vi "List Contents of Azure Container.vi"() -> ()   [LabVIEW 2015]
doc: "Demonstrates how to display the contents of a container for the Azure Blob Service."
uses:
  Core/Azure Credentials.ctl
  Core/NI_Azure_Core.lvlib
  Core/Session/Session.lvclass
  Blob Storage/NI_Azure_Blob.lvlib
panel:
  in  "Access Key":string
  in  "Container Name":string
  in  "Storage Account Name":string
  out "Container Contents":i32(listbox)
  # "Overview: Demonstrates how to display the contents of a container for the Azure Blob Service.\nRequirements: NI Cloud Toolkit for Azure and a registered Microsoft Azure account\nInstructions:\n1. Specify the Storage Account Name and Access Key for your Azure account. You can create an account at http://azure.microsoft.com.\n2. Specify a Container Name for the container you want to inspect.\n3. Run the VI. All of the contents of the specified container will be displayed in the Container Contents indicator."
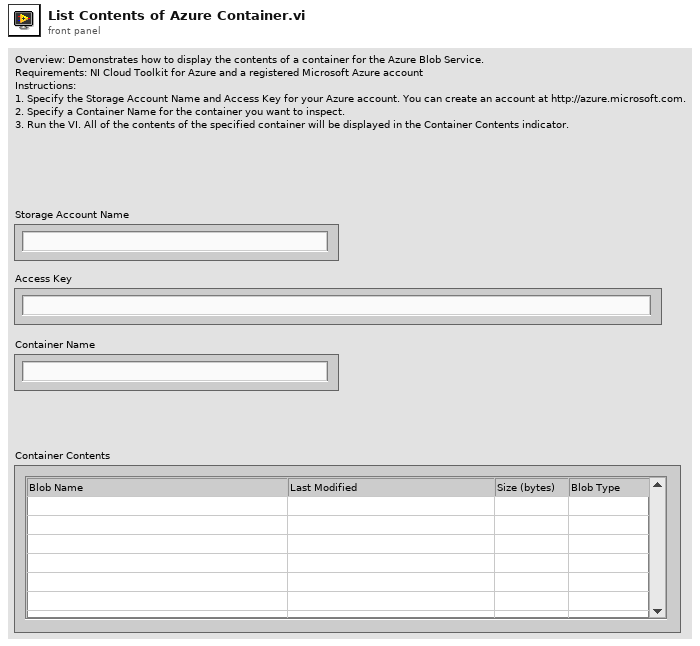
[diagram p1: front panel]
types:
  T1 = typedef "NI_Azure_Core.lvlib/Azure Credentials.ctl" = cluster{"Storage Account Name":string, "Access Key":string}
  T2 = typedef "NI_Azure_Core.lvlib/Name Value Pair.ctl" = cluster{"name":string, "value":string}
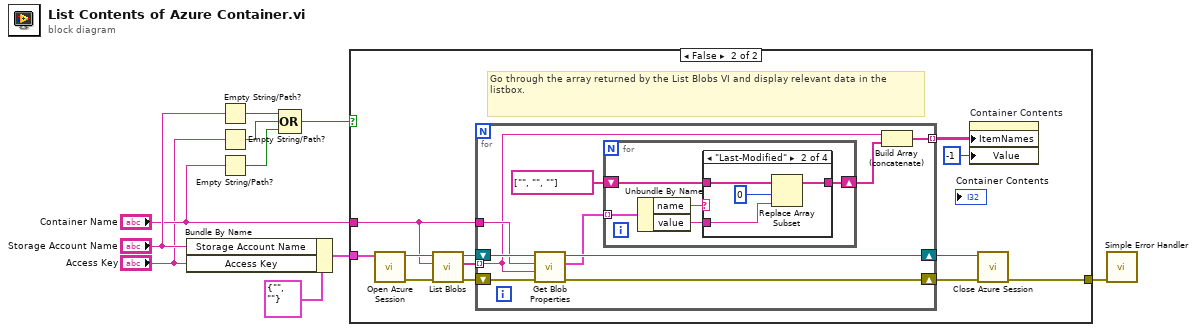
[diagram p0: block diagram]
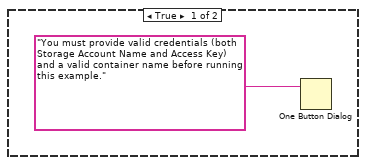
[diagram p2: hidden frame]
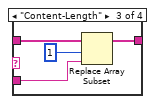
[diagram p4: hidden frame]
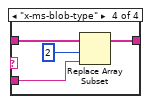
[diagram p5: hidden frame]
diagram:
  n1 = Bundle By Name(cluster=T1 {"Storage Account Name"="", "Access Key"=""} ("Credentials"), "Storage Account Name"="Storage Account Name", "Access Key"="Access Key") -> (w3:T1)
  n2 = Empty String/Path?(string/path="Storage Account Name") -> (empty?=w10:bool)
  n3 = Empty String/Path?(string/path="Access Key") -> (empty?=w9:bool)
  n4 = Empty String/Path?(string/path="Container Name") -> (empty?=w4:bool)
  n5 = Compound Arithmetic op=OR(w10, w9, w4) -> (w7:bool)
  n6 = case shown="False" w7 {
    tunnel: w3 -> [_ w23]
    tunnel: [_ w16] -> w6
    tunnel: "Container Name" -> [_ w14]
    frame True {
      n7 = One Button Dialog(message="You must provide valid credentials (both Storage Account Name and Access Key) and a valid container name before running this example.") -> ()  [unwired: 1 in, 1 out]
    }
    frame False {
      # "Go through the array returned by the List Blobs VI and display relevant data in the listbox."
      n8 = call "Open Azure Session.vi"("Credentials"=w23) -> ("error out"=w22:errorcluster, "Azure Session"=w21:refnum<class "Session.lvclass">)  [unwired: 9 in]
      n9 = call "List Blobs.vi"("error in (no error)"=w22, "Container"=w14, "Azure Session in"=w21) -> ("error out"=w20:errorcluster, "Blobs"=w15:string[], "Azure Session out"=w19:refnum<class "Session.lvclass">)  [unwired: 6 in]
      n10 = for {
        tunnel: w15 -> [w28] mode=indexing
        shift-right: [w29] -> w17
        shift-left: w20 -> [w33]
        shift-right: [w30] -> w18
        shift-left: w19 -> [w32]
        tunnel: w14 -> [w31]
        tunnel: [w27] -> w13 mode=indexing
        n11 = call "Get Blob Properties.vi"("error in (no error)"=w33, "Blob"=w28, "Container"=w31, "Azure Session in"=w32) -> ("error out"=w29:errorcluster, "Blob Properties"=w26:T2[], "Azure Session out"=w30:refnum<class "Session.lvclass">)  [unwired: 5 in]
        n12 = for {
          tunnel: w26 -> [w38] mode=indexing
          shift-right: [w34] -> w25
          shift-left: string[] ["", "", ""] -> [w35]
          n13 = Unbundle By Name(w38) -> ("name"=w37:string, "value"=w36:string)
          n14 = case shown="\"Last-Modified\"" w37 {
            tunnel: w36 -> [_ w41 w45 w49]
            tunnel: w35 -> [w39 w43 w47 w51]
            tunnel: [w39 w42 w46 w50] -> w34
            frame Default {
            }
            frame "Last-Modified" {
              n15 = Replace Array Subset(array=w43, new element=w41, index=0) -> (w42:string[])
            }
            frame "Content-Length" {
              n16 = Replace Array Subset(array=w47, new element=w45, index=1) -> (w46:string[])
            }
            frame "x-ms-blob-type" {
              n17 = Replace Array Subset(array=w51, new element=w49, index=2) -> (w50:string[])
            }
          }
        }
        n18 = Build Array (concatenate)(w28, w25) -> (w27:string[])
      }
      n19 = property on="Container Contents" class="MCListbox (strict)"("ItemNames"=w13, "Value"=-1 ("Container Contents")) -> ()  [unwired: 2 in, 2 out]
      n20 = call "Close Azure Session.vi"("error in (no error)"=w17, "Azure Session"=w18) -> ("error out"=w16:errorcluster)  [unwired: 9 in]
    }
  }
  n21 = call <vilib>:"Simple Error Handler.vi"("error in (no error)"=w6) -> ()  [unwired: 4 in, 5 out]
